vi "Actor Core.vi"(8 "error in":errorcluster, 11 "Controller in":refnum<class "Controller.lvclass">) -> (0 "error out":errorcluster, 3 "Actor out":refnum<class "Actor.lvclass">)   [LabVIEW 2022 SP3, in "Test.lvlib" / "Controller.lvclass"]
doc: "(<B>Filename</B>: Actor Framework.lvlib:Actor.lvclass:Actor Core.vi)\n\nReceives messages to the actor, reacts to them, and initiates any error handling that may shut the actor down.\n\nDescendant classes may override this VI to append parallel tasks for the actor to complete while it handles messages. Overrides use the Call Parent Class Method node."
uses:
  Controller.lvclass
  <vilib>/ActorFramework/Actor/Actor.lvclass
  SubActorOne/SubActorOne.lvclass
  C:/Users/jakub/repos/gh/sw4sys/lv-logging-actor/LoggingActor/Source/LoggingActor/LoggingActor/LoggingActor.lvclass
  C:/Program Files (x86)/National Instruments/LabVIEW 2022/vi.lib/ActorFramework/Actor/Actor.lvclass
  C:/Users/jakub/repos/gh/sw4sys/lv-logging-actor/LoggingActor/Source/Test/Controller/Controller.lvclass
  Gui/Gui/Gui.lvclass
  LoggingActor/LoggingActor/LoggingActor.lvclass
  C:/Users/jakub/repos/gh/sw4sys/lv-logging-actor/LoggingActor/Source/Test/Gui/Gui.lvclass
  C:/Users/jakub/repos/gh/sw4sys/lv-logging-actor/LoggingActor/Source/Test/SubActorOne/SubActorOne.lvclass
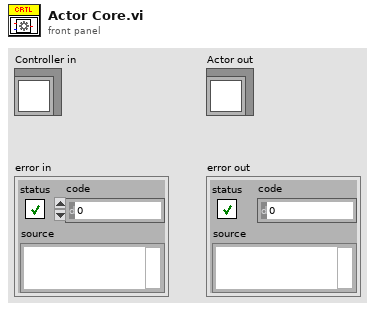
[diagram p1: front panel]
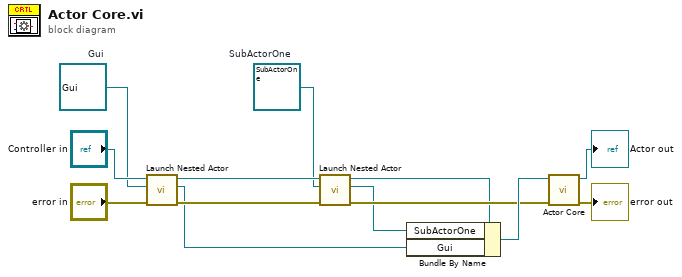
[diagram p0: block diagram]
diagram:
  w2 = refnum<class "Gui.lvclass"> refnum  # Gui
  w3 = refnum<class "SubActorOne.lvclass"> refnum  # SubActorOne
  n1 = call <vilib>:"Launch Nested Actor.vi"("error in (no error)"="error in", "Nested Actor"=w2, "Caller Actor in"="Controller in") -> ("error out"=w10:errorcluster, "Nested Actor's Enqueuer"=w8:refnum<class "Message Enqueuer.lvclass">, "Caller Actor out"=w5:refnum<class "Controller.lvclass">)  [unwired: 6 in]
  n2 = call <vilib>:"Launch Nested Actor.vi"("error in (no error)"=w10, "Nested Actor"=w3, "Caller Actor in"=w5) -> ("error out"=w6:errorcluster, "Nested Actor's Enqueuer"=w1:refnum<class "Message Enqueuer.lvclass">, "Caller Actor out"=w4:refnum<class "Controller.lvclass">)  [unwired: 6 in]
  n3 = Bundle By Name(cluster=w4, "SubActorOne"=w1, "Gui"=w8) -> (w7:refnum<class "Controller.lvclass">)
  n4 = call-parent "Actor Core.vi"("error in"=w6, "Actor in"=w7) -> ("error out"=→"error out":errorcluster, "Actor out"=→"Actor out":refnum<class "Actor.lvclass">)  [unwired: 8 in]
